vi "OP500Z8_OuCrash_P.vi"(2 "Booléen":bool, 3 "in":T1=enum."Scan") -> (0 "OUT":T1=enum."Scan")   [LabVIEW 2020]
uses:
  OP300ZP_state.ctl
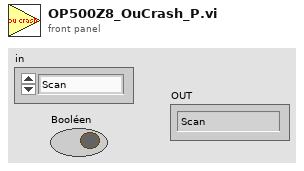
[diagram p1: front panel]
types:
  T1 = typedef "OP300ZP_state.ctl" = enum16{"Null", "Demarrage", "Init", "Scan", "Montage", "Conti", "OCV", "Iso", "Vpack", "DataDyn", "Dessouter", "DataDyn2", "Demontage", "Crash", "Next", "Sealing", "Comext"}
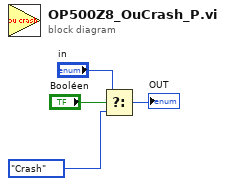
[diagram p0: block diagram]
diagram:
  n1 = Select(t="in", s="Booléen", f=OP300ZP_state."Crash") -> (s? t:f=→"OUT":T1)
